vi "Result.Check if Limit is Numeric.vi"(9 "UL":string, 10 "LL":string, 11 "LimType":T1) -> (1 "UL Num":dbl, 2 "LL Num":dbl, 3 "Is Numeric":bool)   [LabVIEW 2019]
uses:
  Result.Limit Type.ctl
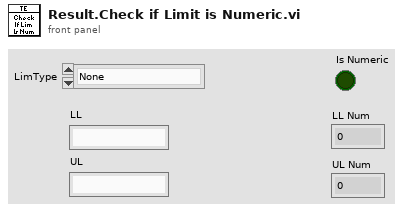
[diagram p1: front panel]
types:
  T1 = typedef "Result.Limit Type.ctl" = enum16{"None", "EQ", "NE", "GT", "LT", "GE", "LE", "GTLT", "GELE", "GELT", "GTLE", "LTGT", "LEGE", "LEGT", "LTGE", "Contains", "NotContains"}
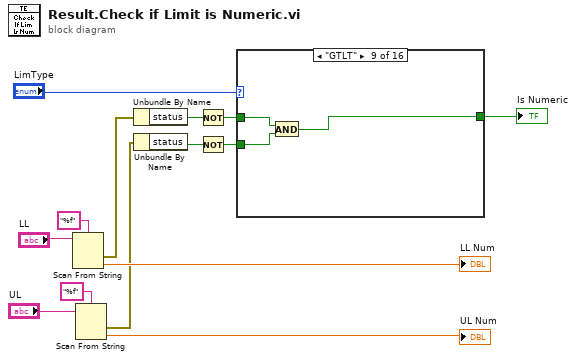
[diagram p0: block diagram]
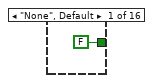
[diagram p2: hidden frame]
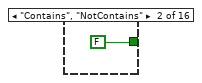
[diagram p3: hidden frame]
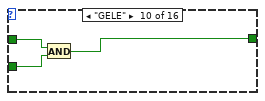
[diagram p10: hidden frame]
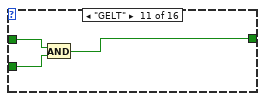
[diagram p11: hidden frame]
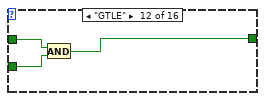
[diagram p12: hidden frame]
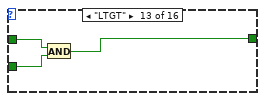
[diagram p13: hidden frame]
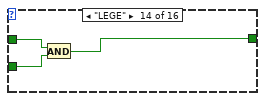
[diagram p14: hidden frame]
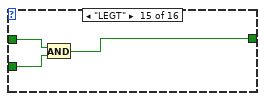
[diagram p15: hidden frame]
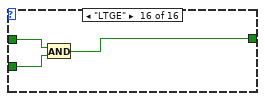
[diagram p16: hidden frame]
diagram:
  n1 = Scan From String(format string="%f", input string="LL") -> (error out=w7:errorcluster, output 1=→"LL Num":dbl)  [unwired: 3 in, 2 out]
  n2 = Scan From String(format string="%f", input string="UL") -> (error out=w6:errorcluster, output 1=→"UL Num":dbl)  [unwired: 3 in, 2 out]
  n3 = Unbundle By Name(w7) -> ("status"=w4:bool)
  n4 = Unbundle By Name(w6) -> ("status"=w3:bool)
  n5 = Not(x=w4) -> (.not. x?=w1:bool)
  n6 = Not(x=w3) -> (.not. x?=w2:bool)
  n7 = case shown="\"GTLT\"" "LimType" {
    tunnel: [FALSE FALSE w17 w18 w19 w20 w21 w22 w23 w26 w29 w32 w35 w38 w41 w44] -> w5
    tunnel: w2 -> [_ _ _ _ _ w20 _ w22 w24 w27 w30 w33 w36 w39 w42 w45]
    tunnel: w1 -> [_ _ w17 w18 w19 _ w21 _ w25 w28 w31 w34 w37 w40 w43 w46]
    frame "None", Default {
    }
    frame "Contains", "NotContains" {
    }
    frame "EQ" {
    }
    frame "NE" {
    }
    frame "GT" {
    }
    frame "LT" {
    }
    frame "GE" {
    }
    frame "LE" {
    }
    frame "GTLT" {
      n8 = And(x=w25, y=w24) -> (x .and. y?=w23:bool)
    }
    frame "GELE" {
      n9 = And(x=w28, y=w27) -> (x .and. y?=w26:bool)
    }
    frame "GELT" {
      n10 = And(x=w31, y=w30) -> (x .and. y?=w29:bool)
    }
    frame "GTLE" {
      n11 = And(x=w34, y=w33) -> (x .and. y?=w32:bool)
    }
    frame "LTGT" {
      n12 = And(x=w37, y=w36) -> (x .and. y?=w35:bool)
    }
    frame "LEGE" {
      n13 = And(x=w40, y=w39) -> (x .and. y?=w38:bool)
    }
    frame "LEGT" {
      n14 = And(x=w43, y=w42) -> (x .and. y?=w41:bool)
    }
    frame "LTGE" {
      n15 = And(x=w46, y=w45) -> (x .and. y?=w44:bool)
    }
  }
  "Is Numeric" <- w5
